vi "Set Rate for Waveform Stream (Custom Rate).vi"(8 "error in (no error)":errorcluster, 10 "custom rate":dbl, 11 "WaveformStreamSpecification in":T1) -> (0 "error out":errorcluster, 3 "WaveformStreamSpecification out":T1)   [LabVIEW 2020, in "NI_VS Waveform Streaming Interface.lvlib"]
doc: "Sets whether to stream waveform values at the same rate the device acquires data or at a custom rate you specify. You must manually select the polymorphic instance to use."
uses:
  <vilib>/NI VeriStand/Execution/WaveformStreaming/NI_VS Waveform Streaming Interface.lvlib
  <vilib>/NI VeriStand/Execution/WaveformStreaming/WaveformStreamSpecification.ctl
  NationalInstruments.VeriStand.ClientAPI
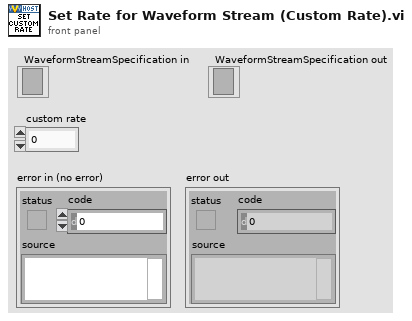
[diagram p1: front panel]
types:
  T1 = typedef "NI_VS Waveform Streaming Interface.lvlib/WaveformStreamSpecification.ctl" = refnum<k24>
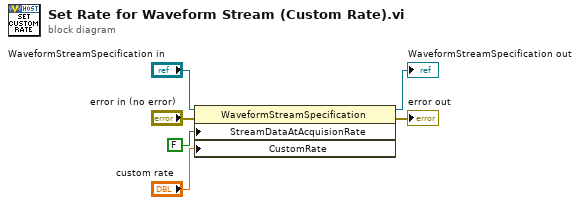
[diagram p0: block diagram]
diagram:
  n1 = property class="WaveformStreamSpecification"(reference="WaveformStreamSpecification in", error in="error in (no error)", "StreamDataAtAcquisionRate"=FALSE, "CustomRate"="custom rate") -> (reference out=→"WaveformStreamSpecification out":T1, error out=→"error out":errorcluster)
